vi "Progress-Bar.vi"(0 "string":string, 1 "Size":i32, 2 "Increment":i32) -> (6 "Prog Bar Ref":refnum<vi>)   [LabVIEW 2013]
panel:
  out "concatenated string":string
  out "Slide":i32(slide) scale=0.0..100.0
  # "%"
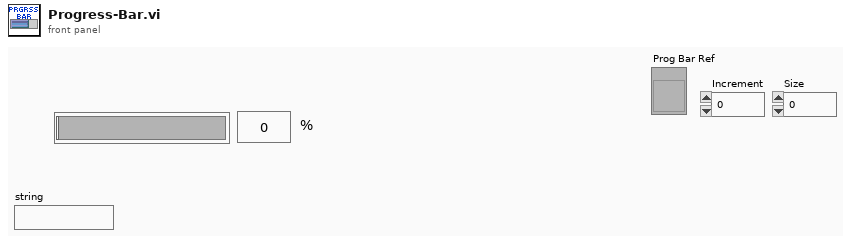
[diagram p1: front panel]
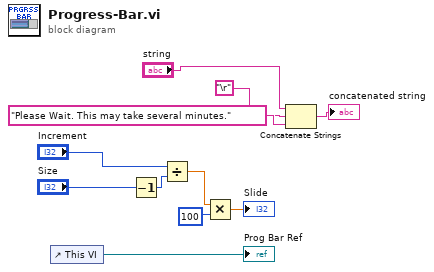
[diagram p0: block diagram]
diagram:
  n1 = control-ref of="This VI"() -> (→"Prog Bar Ref":refnum<vi>)
  n2 = Decrement(x="Size") -> (x-1=w8:i32)
  n3 = Divide(x="Increment", y=w8) -> (x/y=w7:dbl)
  n4 = Multiply(x=w7, y=100) -> (x*y=→"Slide":dbl)
  n5 = Concatenate Strings("string", "\r", "Please Wait. This may take several minutes.") -> (→"concatenated string":string)
